vi "Initialize_Filtering_Settings-4.vi"(1 "Sigma #1":dbl) -> (0 "[OUT] Image Filtering Settings":T1)   [LabVIEW 2017]
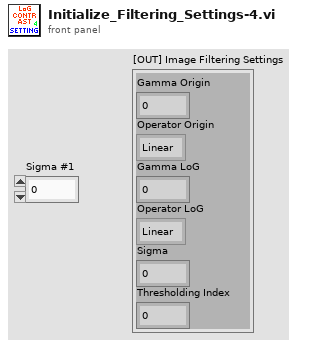
[diagram p1: front panel]
types:
  T1 = cluster{"Gamma Origin":sgl, "Operator Origin":enum32{"Linear", "Log", "Exp", "Square", "Square root", "Power X", "Power 1/X"}, "Gamma LoG":sgl, "Operator LoG":enum32{"Linear", "Log", "Exp", "Square", "Square root", "Power X", "Power 1/X"}, "Sigma":dbl, "Thresholding Index":i8}
  T2 = enum32{"Linear", "Log", "Exp", "Square", "Square root", "Power X", "Power 1/X"}
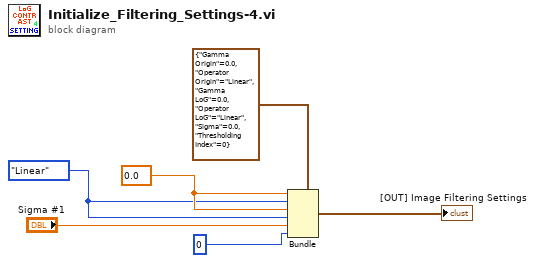
[diagram p0: block diagram]
diagram:
  w5 = T2."Linear" ("Operator 3")
  w6 = sgl 0.0 ("Intensity Increase 3")
  n1 = Bundle(cluster=T1 {"Gamma Origin"=0.0, "Operator Origin"=enum."Linear", "Gamma LoG"=0.0, "Operator LoG"=enum."Linear", "Sigma"=0.0, "Thresholding Index"=0} ("Image Settings"), "Gamma Origin"=w6, "Operator Origin"=w5, "Gamma LoG"=w6, "Operator LoG"=w5, "Sigma"="Sigma #1", "Thresholding Index"=i8 0 ("Index for \nthresholding")) -> (→"[OUT] Image Filtering Settings":T1)
